vi "ANC300_Preferences.vi"(0 "ANC300 Communication Port In":refnum<visa-resource-name>, 1 "connection ID in":refnum<k5>, 2 "Axis":u8=1 min=1 max=7, 3 "value in":dbl=10.0 min=0.0 format="%.1f", 4 "parameter":string(combo)="v ", 5 "error in":T1, 6 "set / get":bool=TRUE, 7 "Time to wait [ms]":u32=200) -> (12 "command string":string, 13 "data out":string, 14 "ANC300 Communication Port Out":refnum<visa-resource-name>, 15 "connection ID out":refnum<k5>, 16 "value out":dbl, 17 "unit":string, 18 "transfer ok":bool, 19 "error out":T1)   [LabVIEW 2022 SP3]
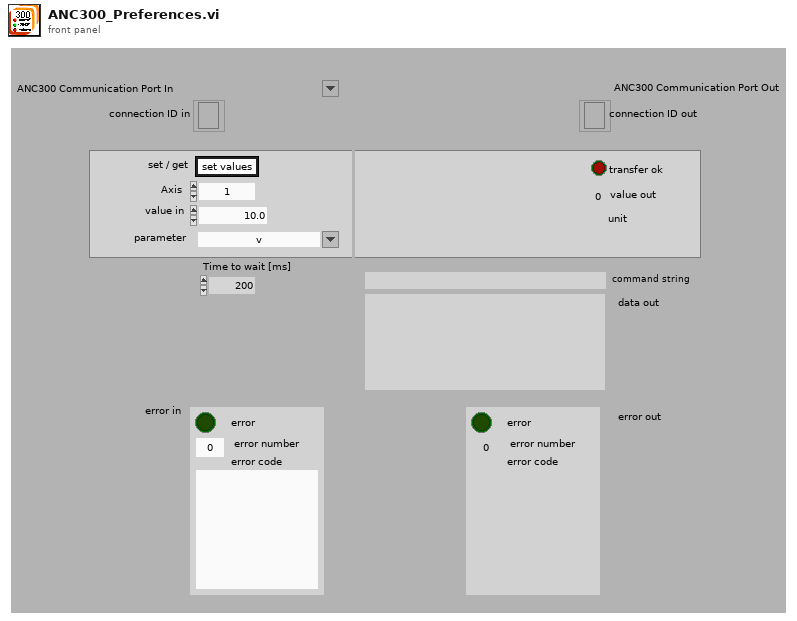
[diagram p1: front panel]
types:
  T1 = cluster{"error ":bool, "error number":i32, "error code":string}
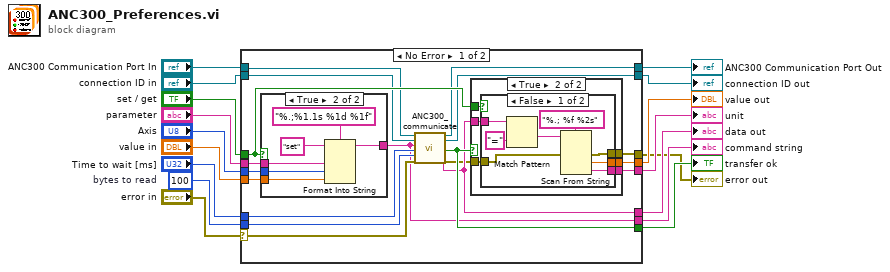
[diagram p0: block diagram]
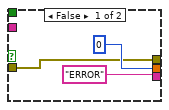
[diagram p2: hidden frame]
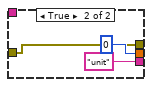
[diagram p3: hidden frame]
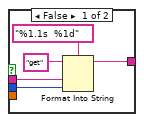
[diagram p4: hidden frame]
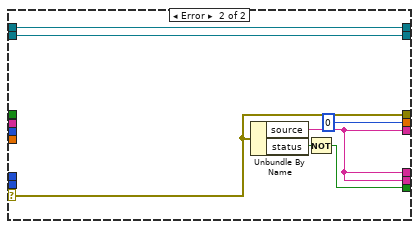
[diagram p5: hidden frame]
diagram:
  w10 = 100  # bytes to read
  n1 = case shown="No Error" "error in" {
    selector: "error in" -> [w23 w67]
    tunnel: "parameter" -> [w35 _]
    tunnel: "Axis" -> [w34 _]
    tunnel: "value in" -> [w33 _]
    tunnel: "set / get" -> [w32 _]
    tunnel: "ANC300 Communication Port In" -> [w31 w73]
    tunnel: "connection ID in" -> [w30 w72]
    tunnel: "Time to wait [ms]" -> [w29 _]
    tunnel: w10 -> [w28 _]
    tunnel: [w27 0] -> w6
    tunnel: [w26 w68] -> w5
    tunnel: [w25 w73] -> w8
    tunnel: [w24 w72] -> w7
    tunnel: [w22 w69] -> w2
    tunnel: [w21 w68] -> w4
    tunnel: [w20 w68] -> w3
    tunnel: [w18 w67] -> w1
    frame No Error {
      n2 = case shown="True" w32 {
        tunnel: w34 -> [w56 w64]
        tunnel: w35 -> [w57 w63]
        tunnel: w33 -> [_ w62]
        tunnel: [w58 w61] -> w21
        frame False {
          n3 = Format Into String(format string="%1.1s  %1d", initial string="get", w57, w56) -> (resulting string=w58:string)  [unwired: 1 in, 1 out]
        }
        frame True {
          n4 = Format Into String(format string="%.;%1.1s %1d %1f", initial string="set", w63, w64, w62) -> (resulting string=w61:string)  [unwired: 1 in, 1 out]
        }
      }
      n5 = call "ANC300_communicate.vi"("ANC300 Communication Port In"=w31, "connection ID in"=w30, "commando string"=w21, "Time to wait [ms]"=w29, "bytes to read"=w28, "error in"=w23) -> ("ANC300 Communication Port Out"=w25:refnum<visa-resource-name>, "connection ID out"=w24:refnum<k5>, "read data"=w20:string, "transfer ok"=w22:bool, "error out"=w19:T1)  [unwired: 9 in]
      n6 = case shown="True" w22 {
        tunnel: ["ERROR" w44] -> w26
        tunnel: [0 w43] -> w27
        tunnel: w20 -> [_ w42]
        tunnel: w32 -> [_ w41]
        tunnel: w19 -> [w36 w40]
        tunnel: [w36 w39] -> w18
        frame False {
        }
        frame True {
          n7 = case shown="False" w41 {
            tunnel: w42 -> [w49 _]
            tunnel: [w48 u8 0] -> w43
            tunnel: [w47 "unit" ("data out")] -> w44
            tunnel: w40 -> [w46 w53]
            tunnel: [w45 w53] -> w39
            frame False {
              n8 = Match Pattern(string=w49, regular expression="=") -> (after substring=w52:string)  [unwired: 1 in, 3 out]
              n9 = Scan From String(format string="%.; %f %2s", input string=w52, error in=w46) -> (error out=w45:errorcluster, output 1=w48:dbl, output 2=w47:string)  [unwired: 3 in, 2 out]
            }
            frame True {
            }
          }
        }
      }
    }
    frame Error {
      n10 = Unbundle By Name(w67) -> ("source"=w68:string, "status"=w70:bool)
      n11 = Not(x=w70) -> (.not. x?=w69:bool)
    }
  }
  "data out" <- w3
  "connection ID out" <- w7
  "error out" <- w1
  "command string" <- w4
  "value out" <- w6
  "unit" <- w5
  "transfer ok" <- w2
  "ANC300 Communication Port Out" <- w8
